vi "_save_csv_EVM_LitePoint_JIO.vi"(7 "delimiter (\\t)":string="SingleCh_", 11 "array in":string[][](array[string])) -> (3 "FileName":string)   [LabVIEW 2023]
uses:
  <vilib>/Utility/file.llb/Write Delimited Spreadsheet (string).vi
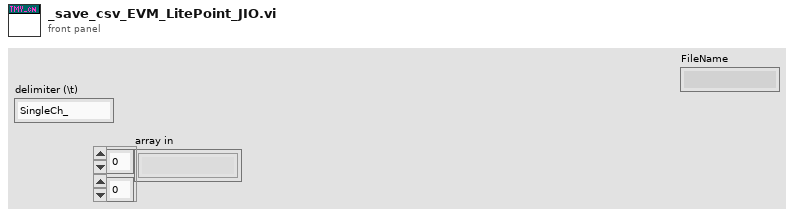
[diagram p1: front panel]
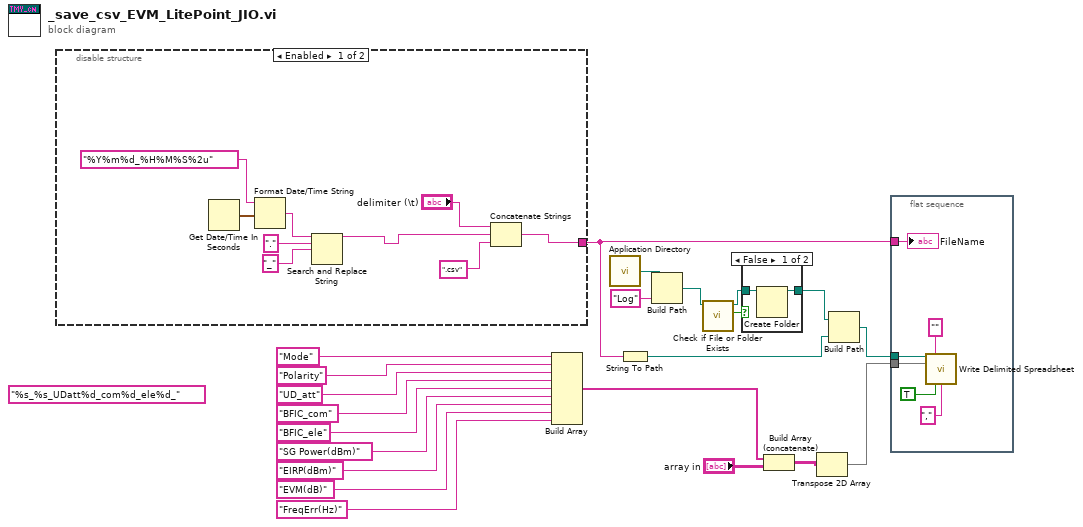
[diagram p0: block diagram]
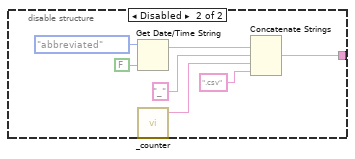
[diagram p3: hidden frame]
diagram:
  (unwired) "%s_%s_UDatt%d_com%d_ele%d_" ("format string")
  n1 = disable-structure shown="Enabled" {
    disable-tunnel: [w30 w32] -> w19
    frame Enabled {
      n2 = Get Date/Time In Seconds() -> (seconds since 1Jan1904=w28:timestamp)
      n3 = Format Date/Time String(time format string (%c)="%Y%m%d_%H%M%S%2u", seconds (now)=w28) -> (date/time string=w26:string)  [unwired: 1 in]
      n4 = Search and Replace String(input string=w26, search string=".", replace string="_") -> (result string=w23:string)  [unwired: 5 in, 3 out]
      n5 = Concatenate Strings("delimiter (\\t)", w23, ".csv" ("delimiter (\\t)")) -> (w30:string)
    }
    frame Disabled {
      n6 = Get Date/Time String(date format (0)=enum16{"short", "long", "abbreviated"}."abbreviated", want seconds? (F)=FALSE) -> (date string=w39:string)  [unwired: 1 in, 1 out]
      n7 = call "_counter.vi"() -> ("out_count"=w33:string)  [unwired: 5 in]
      n8 = Concatenate Strings(w39, "_" ("delimiter (\\t)"), w33, ".csv" ("delimiter (\\t)")) -> (w32:string, w34:string)
    }
  }
  n9 = Build Array("Mode", "Polarity", "UD_att", "BFIC_com", "BFIC_ele", "SG Power(dBm)", "EIRP(dBm)", "EVM(dB)", "FreqErr(Hz)") -> (w13:string[])
  n10 = call <vilib>:"Application Directory.vi"() -> ("Application Directory"=w18:path)
  n11 = String To Path(string=w19) -> (path=w21:path)
  n12 = Build Path(base path=w18, name or relative path="Log") -> (appended path=w15:path)
  n13 = call <vilib>:"Check if File or Folder Exists.vi"("path"=w15) -> ("file or folder exists?"=w17:bool, "dup path"=w16:path)  [unwired: 8 in, 1 out]
  n14 = case shown="False" w17 {
    tunnel: w16 -> [w41 w42]
    tunnel: [w40 w42] -> w14
    frame False {
      n15 = Create Folder(path (use dialog)=w41) -> (created path=w40:path)  [unwired: 2 in, 2 out]
    }
    frame True {
    }
  }
  n16 = Build Array (concatenate)(w13, "array in") -> (w10:string[][])
  n17 = Transpose 2D Array(2D array=w10) -> (transposed array=w12:string[][])
  n18 = Build Path(base path=w14, name or relative path=w21) -> (appended path=w20:path)
  n19 = flat-sequence {
    tunnel: w20 -> [w47]
    tunnel: w19 -> [w45]
    tunnel: w12 -> [w43]
    frame #0 {
      n20 = call-poly <vilib>:"Write Delimited Spreadsheet.vi"("file path (dialog if empty)"=w47, "format (%s)"="" ("format (%.3f)"), "2D data"=w43, "transpose? (no:F)"=TRUE, "delimiter (\\t)"="," ("delimiter (\\t)")) -> ()  [unwired: 9 in, 2 out]
      "FileName" <- w45
    }
  }
